vi "ConfigureMeasurement_DMM2831E.vi"(4 "error in (no error)":errorcluster, 6 "Function (0: DC Volts)":u16(ring) items=["DC Volts", "AC Volts", "AC+DC Volts", "DC Current", "AC Current", "AC+DC Current", "2-Wire Resistance", "Frequency", "Period", "Diode", "Continuity"], 7 "Instrument In":refnum<visa-resource-name>) -> (0 "error out":errorcluster, 1 "Instrument Out":refnum<visa-resource-name>)   [LabVIEW 2023]
uses:
  <instrlib>/BK Precision 5491B/BK Precision 5491B.lvlib
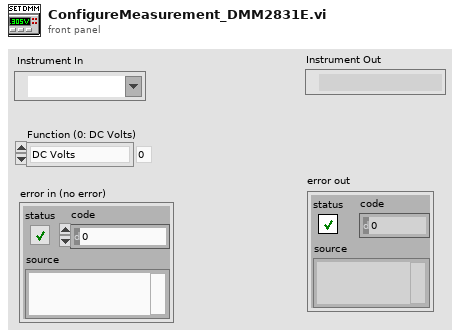
[diagram p1: front panel]
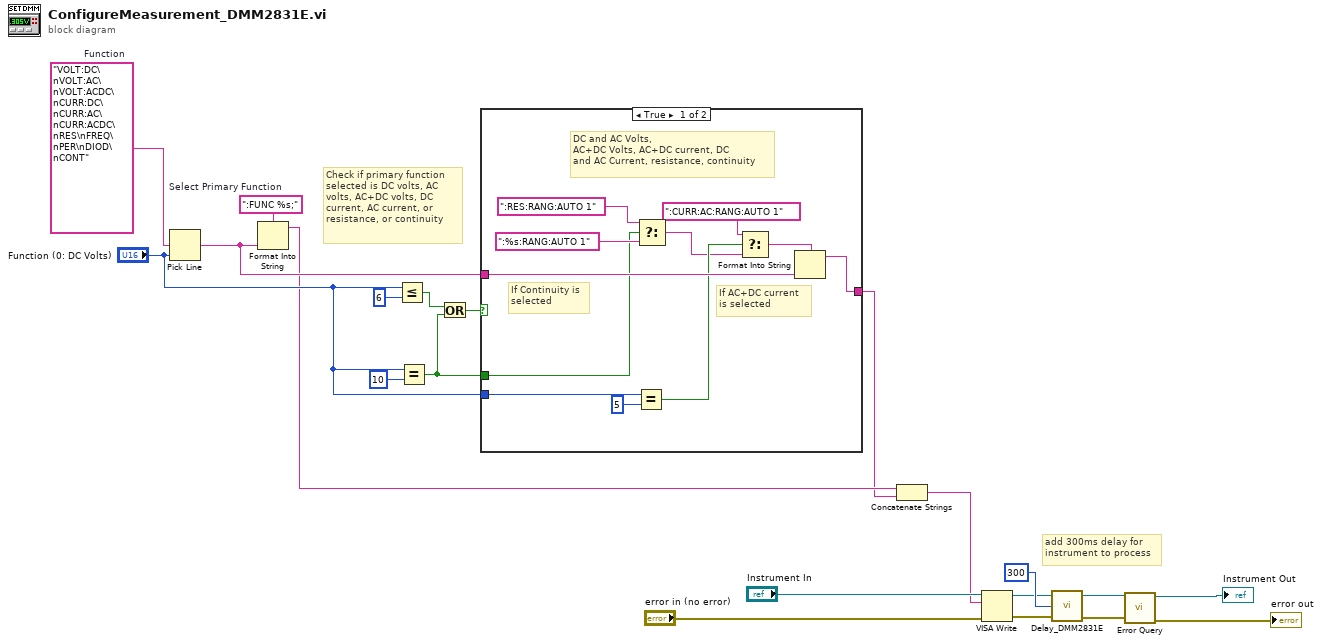
[diagram p0: block diagram]
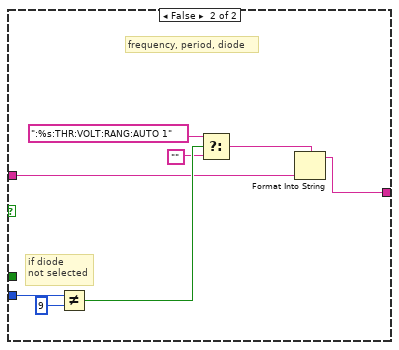
[diagram p2: hidden frame]
diagram:
  w20 = ":FUNC %s;"  # Select Primary Function
  w21 = "VOLT:DC\nVOLT:AC\nVOLT:ACDC\nCURR:DC\nCURR:AC\nCURR:ACDC\nRES\nFREQ\nPER\nDIOD\nCONT"  # Function
  # "add 300ms delay for\ninstrument to process"
  # "Check if primary function\nselected is DC volts, AC\nvolts, AC+DC volts, DC\ncurrent, AC current, or\nresistance, or continuity"
  n1 = Pick Line(multi-line string=w21, line index="Function (0: DC Volts)") -> (output string=w19:string)  [unwired: 1 in]
  n2 = Format Into String(format string=w20, w19) -> (resulting string=w3:string)  [unwired: 2 in, 1 out]
  n3 = Less Or Equal?(x="Function (0: DC Volts)", y=u16 6) -> (x <= y?=w15:bool)
  n4 = Equal?(x="Function (0: DC Volts)", y=u16 10) -> (x = y?=w14:bool)
  n5 = Or(x=w15, y=w14) -> (x .or. y?=w16:bool)
  n6 = case shown="True" w16 {
    tunnel: w19 -> [w32 w34]
    tunnel: [w31 w33] -> w2
    tunnel: w14 -> [w28 _]
    tunnel: "Function (0: DC Volts)" -> [w26 w40]
    frame True {
      # "If AC+DC current\nis selected"
      # "If Continuity is\nselected"
      # "DC and AC Volts,\nAC+DC Volts, AC+DC current, DC\nand AC Current, resistance, continuity"
      n7 = Equal?(x=w26, y=u16 5) -> (x = y?=w25:bool)
      n8 = Select(t=":RES:RANG:AUTO 1", s=w28, f=":%s:RANG:AUTO 1") -> (s? t:f=w24:string)
      n9 = Select(t=":CURR:AC:RANG:AUTO 1", s=w25, f=w24) -> (s? t:f=w22:string)
      n10 = Format Into String(format string=w22, w32) -> (resulting string=w31:string)  [unwired: 2 in, 1 out]
    }
    frame False {
      # "if diode\nnot selected"
      # "frequency, period, diode"
      n11 = Not Equal?(x=w40, y=u16 9) -> (x != y?=w38:bool)
      n12 = Select(t=":%s:THR:VOLT:RANG:AUTO 1", s=w38, f="") -> (s? t:f=w35:string)
      n13 = Format Into String(format string=w35, w34) -> (resulting string=w33:string)  [unwired: 2 in, 1 out]
    }
  }
  n14 = Concatenate Strings(w3, w2) -> (w1:string)
  n15 = VISA Write(VISA resource name="Instrument In", write buffer=w1, error in (no error)="error in (no error)") -> (VISA resource name out=w5:refnum<visa-resource-name>, error out=w6:errorcluster)  [unwired: 1 out]
  n16 = call "Delay_DMM2831E.vi"("error in (no error)"=w6, "Delay Time (0)"=u32 300, "Instrument In"=w5) -> ("error out"=w9:errorcluster, "Instrument Out"=w8:refnum<visa-resource-name>)
  n17 = call <instrlib>:"Error Query.vi"("error in (no error)"=w9, "VISA resource name"=w8) -> ("error out"=→"error out":errorcluster, "VISA resource name out"=→"Instrument Out":refnum<visa-resource-name>)  [unwired: 7 in, 1 out]
